vi "STORE_OUTPUT.vi"(9 "CURRENT_YEAR_DATA":string, 10 "ECODE 2":string, 11 "connection reference":T1) -> ()   [LabVIEW 2015]
uses:
  Controls/ITEM_CODE_CLUSTER.ctl
  <vilib>/addons/database/Connection.llb/Conn ObjectReference.ctl
  <vilib>/Utility/miscctls.llb/LVRowAndColumnUnsignedTypeDef.ctl
  Controls/STORE_OUTPUT_NO_CLUSTER.ctl
  Controls/ITEM_INFORMATION_CLUSTER.ctl
  Controls/Print_Data.ctl
  <vilib>/addons/database/Connection.llb/Conn Execute.vi
  <vilib>/addons/database/Recordset.llb/Rec Destroy - Connection.vi
  <vilib>/addons/database/_DB Variant To Data/Database Variant To Data.xnode
  <vilib>/addons/database/NI_Database_API.lvlib
  <vilib>/addons/database/Connection.llb/DB Tools Open Connec (String).vi
panel:
  in  "BALANCE_PRINT":bool
  in  "Print Button":bool
  out "FIFO_ARRAY":T2[](array[typedef])
  out "Location":string
  out "Lot Maker":string
  out "Maker Code":string
  out "Invoice Date":timestamp format="%<%d/%m/%Y>T"
  out "Invoice No.":string
  in  "Excle Path":path
  in  "BUTTON_EXIT":bool
  in  "BUTTON_INPUT":bool
  out "Unit 2":string
  in  "Quantity (F2)":dbl
  out "Item Code":string
  out "FIFO":string
  in  "QR Code (F3)":string
  out "Maker":string
  out "Part Name":string
  out "Product":string
  out "ECODE":string
  in  "Output Date":timestamp format="%<%d/%m/%Y>T"
  out "Output No.":string
  out "Table":string[][](table)
  # "OUTPUT MATERIAL"
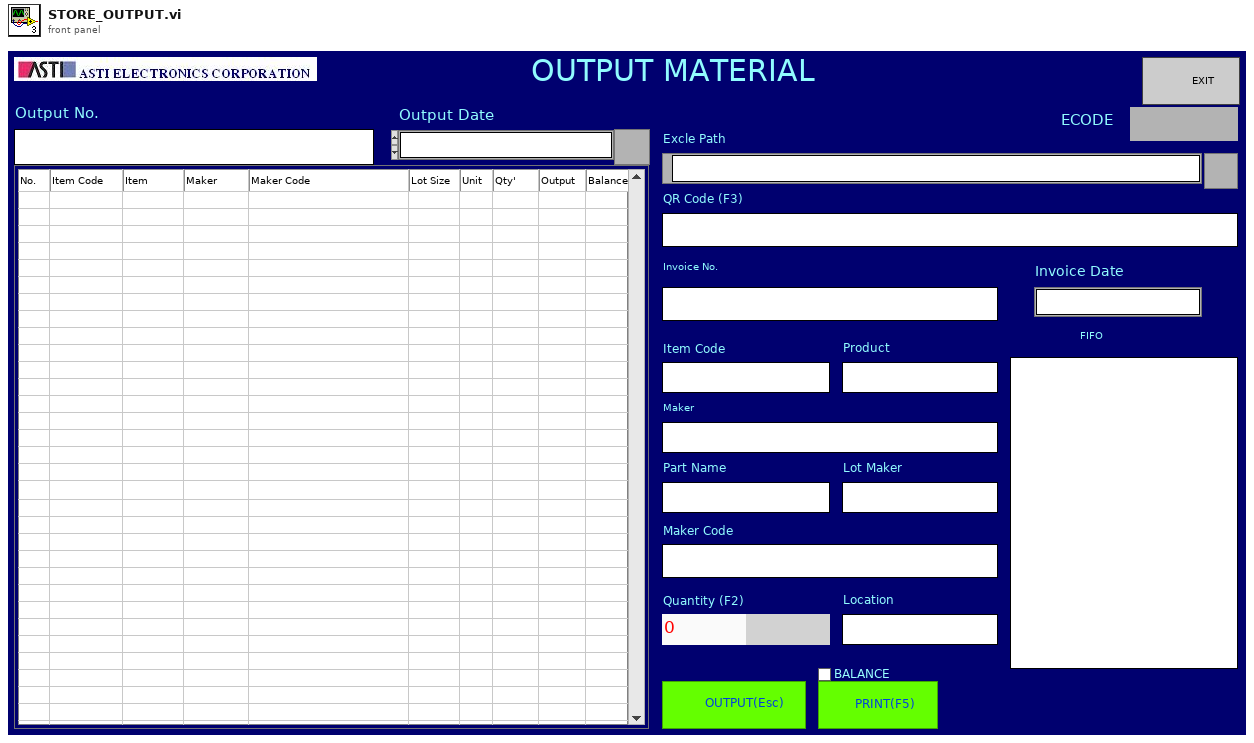
[diagram p1: front panel]
types:
  T1 = typedef "NI_Database_API.lvlib/Conn ObjectReference.ctl" = refnum<k1>
  T2 = typedef "ITEM_CODE_CLUSTER.ctl" = cluster{"ITEM_CODE":string, "INVOICE_NO":string, "INVOICE_DATE":timestamp, "LOT_MAKER":string, "QUANTITY":dbl, "INVOICE_ECODE":string, "INPUT_NO":string, "INPUT_DATE":timestamp, "INPUT_ECODE":string, "LINEBACK_NO":string, "LINEBACK_DATE":timestamp, "LINEBACK_ECODE":string, "OUTPUT_NO":string, "OUTPUT_DATE":timestamp, "OUTPUT_ECODE":string, "DESTINATION":string}
  T3 = typedef "LVRowAndColumnUnsignedTypeDef.ctl" = cluster{"Row":u32, "Column":u32}
  T4 = typedef "STORE_OUTPUT_NO_CLUSTER.ctl" = cluster{"NO":dbl, "ITEM_CODE":string, "ITEM":string, "MAKER":string, "MAKER_CODE":string, "LOT_SIZE":dbl, "UNIT":string, "QUANTITY":dbl, "INPUT":dbl, "BALANCE":dbl, "DESTINATION":string, "OUTPUT_NO":string}
  T5 = cluster{"start (-1, -1)":cluster{"row":i32, "column":i32}, "end (-1, -1)":cluster{"row":i32, "column":i32}}
  T6 = cluster{"OUTPUT_NO":string, "OUTPUT_DATE":timestamp, "ECODE":string}
  T7 = typedef "ITEM_INFORMATION_CLUSTER.ctl" = cluster{"PRODUCT":string, "ITEM_CODE":string, "PART_NAME":string, "MAKER":string, "PART_NO":string, "LOT_SIZE":dbl, "UNIT":string, "LENGTH-OFFSET":string, "BARCODE":string, "PROCESS":string, "INVENTORY_LOCAL":string, "TARE":dbl, "SAMPLE":dbl}
  T8 = typedef "Print_Data.ctl" = cluster{"QR_code Text":string, "Lot Maker":string, "Item Code (F3)":string, "date/time string":string, "Invoice No.":string, "Maker":string, "Part No.(F2) ":string, "Location":string, "Product":string, "Qty":string, "ECODE":string}
  T9 = typedef "NI_Database_API.lvlib/Rec ObjectReference.ctl" = refnum<k1>
  T10 = cluster{"Output No.":string, "seconds since 1Jan1904":timestamp, "ECODE":string, "DESTINATION":string}
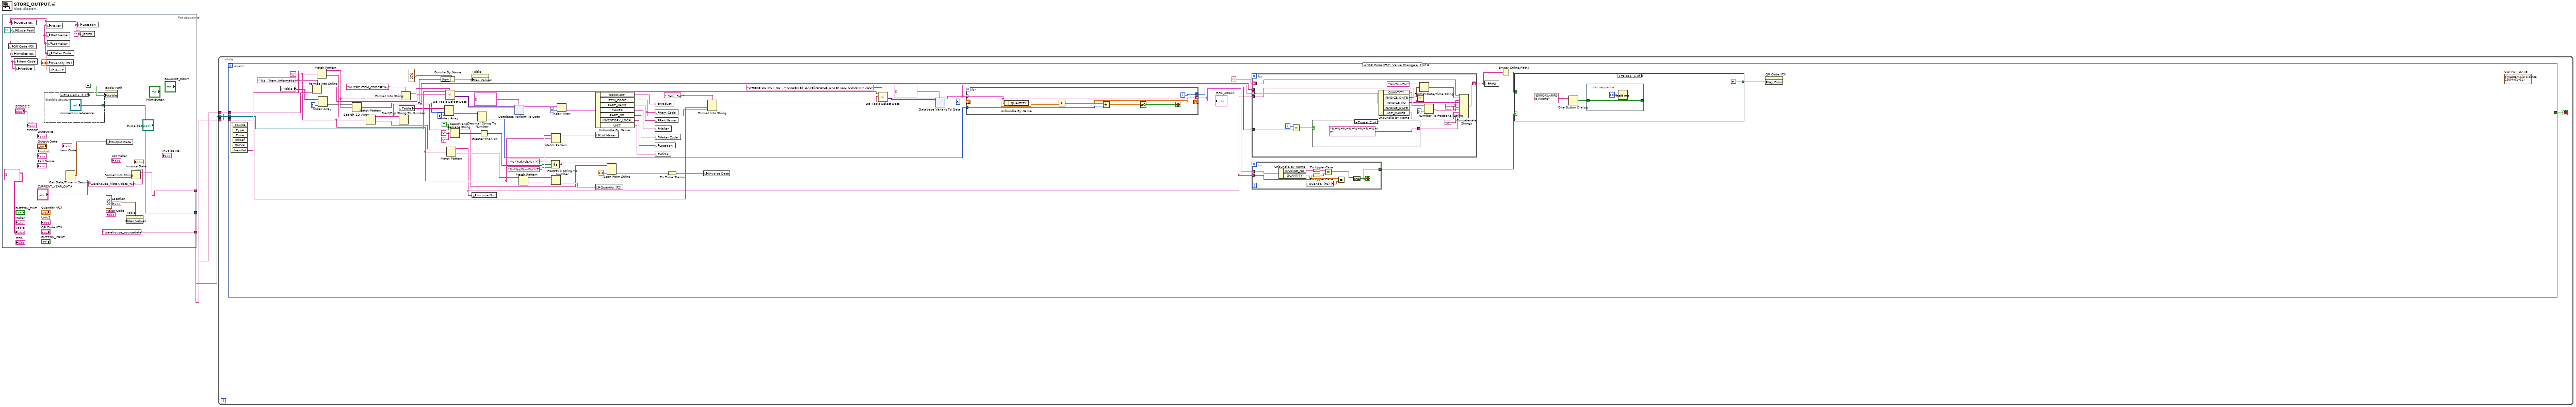
[diagram p0: block diagram]
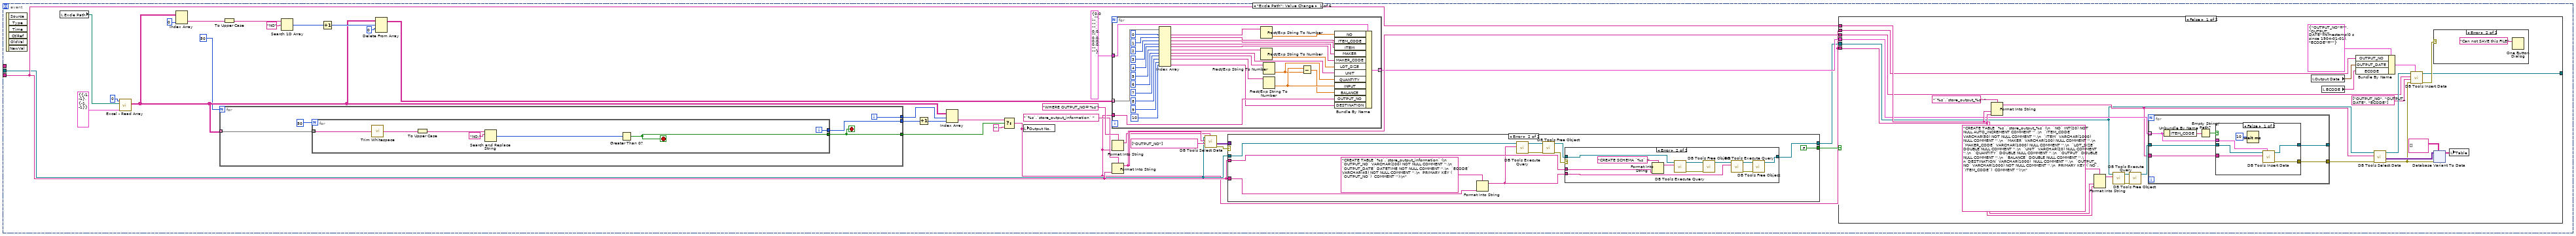
[diagram p2: hidden frame]
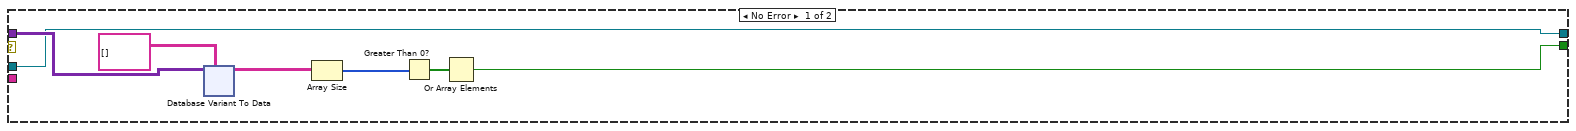
[diagram p3: hidden frame]
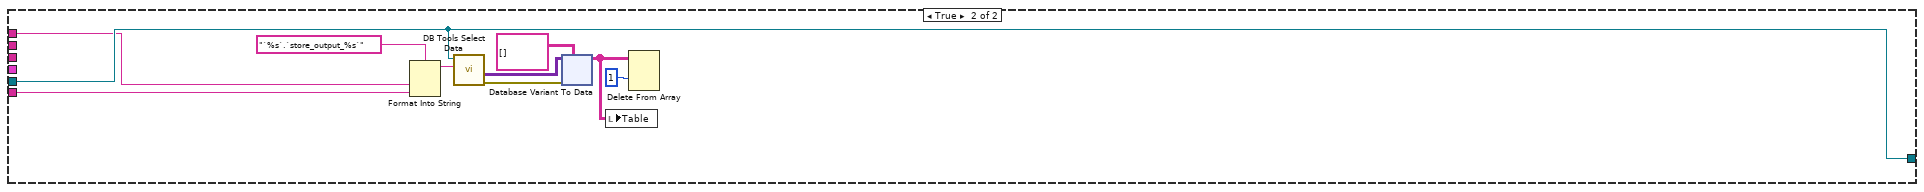
[diagram p7: hidden frame]
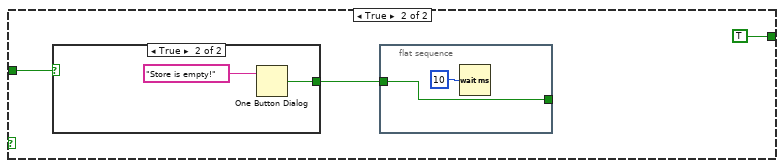
[diagram p8: hidden frame]
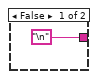
[diagram p10: hidden frame]
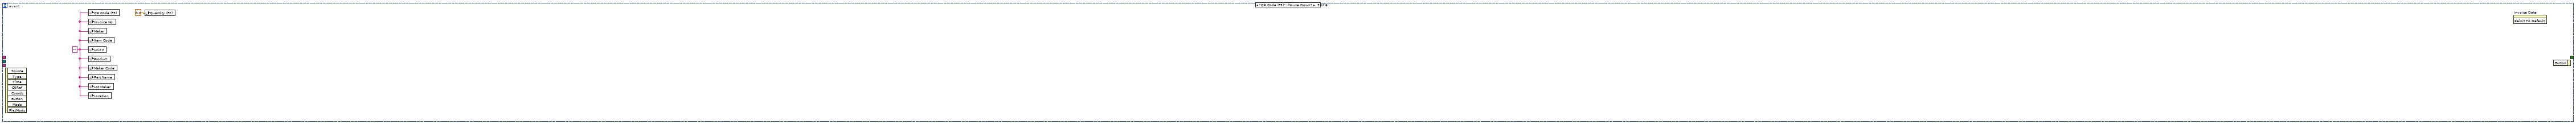
[diagram p11: hidden frame]
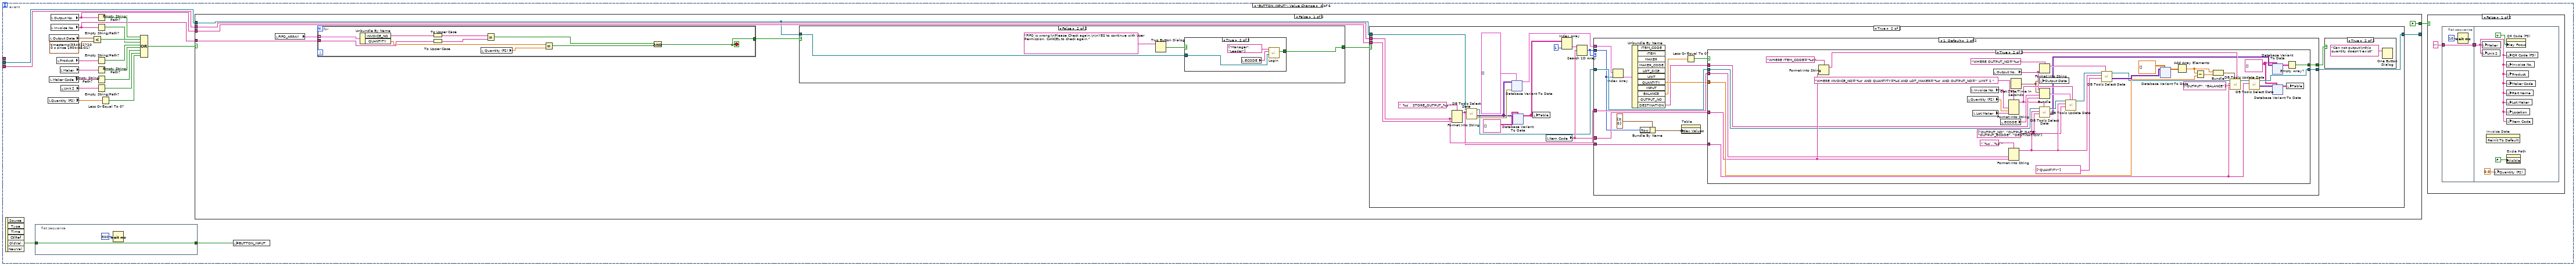
[diagram p12: hidden frame]
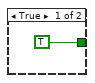
[diagram p14: hidden frame]
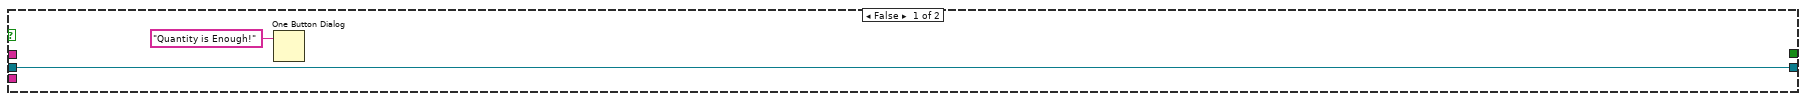
[diagram p18: hidden frame]
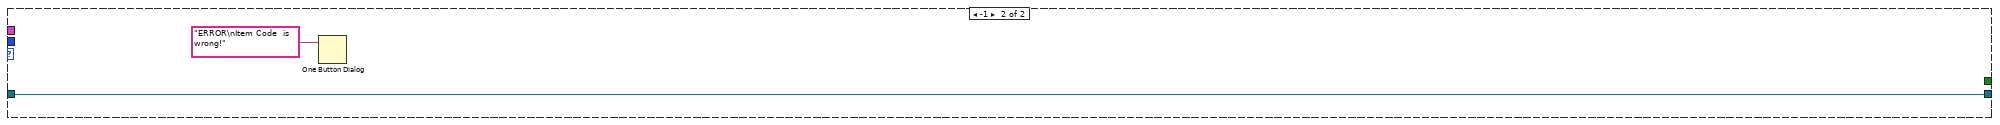
[diagram p19: hidden frame]
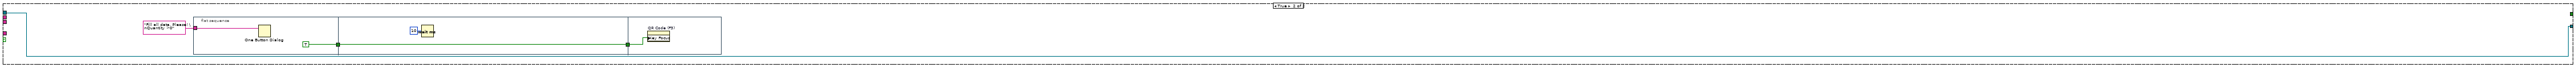
[diagram p20: hidden frame]
diagram:
  n1 = flat-sequence {
    tunnel: [w16] -> w3
    tunnel: [w14] -> w2
    tunnel: ["warehouse_sourcedata" ("table")] -> w1
    frame #0 {
      w12 = "" ("FIFO")
      n2 = local write "QR Code (F3)"(w12) -> ()
      n3 = local write "Invoice No."(w12) -> ()
      n4 = local write "Output No."(w12) -> ()
      n5 = local write "Excle Path"(path "" ("Excle Path")) -> ()
      n6 = local write "Item Code"(w12) -> ()
      n7 = local write "Product"(w12) -> ()
      n8 = disable-structure shown="Enabled" {
        disable-tunnel: [w17 "connection reference"] -> w16
        frame Disabled {
          n9 = call-poly <vilib>:"DB Tools Open Connection.vi"("password"="871994" ("userID"), "userID"="hoangbao2106", "connection information"="Database" ("userID")) -> ("connection reference"=w17:T1)  [unwired: 5 in, 1 out]
        }
        frame Enabled {
        }
      }
      n10 = local write "Maker"(w12) -> ()
      n11 = local write "Part Name"(w12) -> ()
      n12 = local write "Quantity (F2)"(0.0 ("Quantity")) -> ()
      n13 = local write "Lot Maker"(w12) -> ()
      n14 = local write "Maker Code"(w12) -> ()
      n15 = local write "Unit 2"(w12) -> ()
      n16 = Get Date/Time In Seconds() -> (seconds since 1Jan1904=w9:timestamp)
      n17 = local write "Location"(w12) -> ()
      n18 = local write "FIFO"(w12) -> ()
      n19 = property on="Excle Path" class="Path"("Visible"=TRUE) -> ()  [unwired: 2 in, 2 out]
      n20 = local write "Output Date"(w9) -> ()
      n21 = property on="Table" class="Tbl (strict)"("Index Values"=T3 {"Row"=0, "Column"=0}) -> ()  [unwired: 2 in, 2 out]
      n22 = Format Into String(format string="warehouse_historydata_%s" ("table"), "CURRENT_YEAR_DATA") -> (resulting string=w14:string)  [unwired: 2 in, 1 out]
      "Table" <- string[][] []
      "ECODE" <- "ECODE 2"
    }
  }
  n23 = while {
    tunnel: w3 -> [w24]
    tunnel: w2 -> [w23]
    tunnel: w1 -> [w22]
    stop <- w25 stop-if-true
    n24 = event shown="[1] \"QR Code (F3)\": Value Change" {
      selector: _ -> [_ _ _ _ _ _]
      dyn-events: _ -> [_ _ _ _ _ _]
      timeout: _ -> [_ _ _ _ _ _]
      tunnel: [_ _ _ _ _ TRUE] -> w25
      tunnel: w24 -> [w28 w377 _ w1411 _ _]
      tunnel: w23 -> [w29 w360 _ w1410 _ _]
      tunnel: w22 -> [_ w375 _ _ _ _]
      event "Excle Path": Value Change {
        n25 = event-data() -> ()  [unwired: 1 in, 6 out]
        n26 = local read "Excle Path"() -> (w30:path)
        n27 = call "Excel - Read Array.vi"("Cluster"=T5 {"start (-1, -1)"={"row"=-1, "column"=-1}, "end (-1, -1)"={"row"=-1, "column"=-1}}, "Path"=w30, "worksheet index (0)"=0) -> ("Element 1"=w43:string[][])  [unwired: 5 in, 1 out]
        n28 = Index Array(array=w43, index (col)=0 ("disabled index (col)")) -> (element=w41:string[])  [unwired: 1 in]
        n29 = for {
          N: 50 -> [_]
          tunnel: w43 -> [w306] mode=indexing
          tunnel: [w305] -> w36
          tunnel: [w303] -> w34
          tunnel: [w302] -> w33
          i -> [w305]
          stop <- w302 stop-if-true
          n30 = for {
            N: 50 -> [_]
            tunnel: w306 -> [w312] mode=indexing
            tunnel: [w307] -> w302
            tunnel: [w313] -> w303
            i -> [w313]
            stop <- w307 stop-if-true
            n31 = call <vilib>:"Trim Whitespace.vi"("string"=w312) -> ("trimmed string"=w311:string)  [unwired: 1 in]
            n32 = To Upper Case(1:w311) -> (0:w310:string)
            n33 = Search and Replace String(input string=w310, search string="NO:" ("y")) -> (number of replacements=w308:i32)  [unwired: 6 in, 3 out]
            n34 = Greater Than 0?(x=w308) -> (x > 0?=w307:bool)
          }
        }
        n35 = To Upper Case(1:w41) -> (0:w42:string[])
        n36 = Search 1D Array(1D array=w42, element="NO") -> (index of element=w44:i32)  [unwired: 1 in]
        n37 = Increment(x=w44) -> (x+1=w45:i32)
        n38 = Delete From Array(array=w43, length=w45, index (row)=0) -> (array with subset deleted=w55:string[][])  [unwired: 1 in, 1 out]
        n39 = Increment(x=w34) -> (x+1=w35:i32)
        n40 = Index Array(array=w43, index (row)=w36, index (col)=w35) -> (element=w37:string)
        n41 = Select(t=w37, s=w33, f="") -> (s? t:f=w27:string)
        n42 = local write "Output No."(w27) -> ()
        n43 = for {
          tunnel: w55 -> [w87] mode=indexing
          tunnel: T4 {"NO"=0.0, "ITEM_CODE"="", "ITEM"="", "MAKER"="", "MAKER_CODE"="", "LOT_SIZE"=0.0, "UNIT"="", "QUANTITY"=0.0, "INPUT"=0.0, "BALANCE"=0.0, "DESTINATION"="", "OUTPUT_NO"=""} -> [w88]
          tunnel: [w65] -> w57 mode=indexing
          tunnel: w27 -> [w64]
          n44 = Index Array(array=w87, index #1=0 ("index"), index #2=1 ("index"), index #3=2 ("index"), index #4=3 ("index"), index #5=4 ("index"), index #6=5 ("index"), index #7=6 ("index"), index #8=7 ("index"), index #9=8 ("index"), index #10=9 ("index"), index #11=10 ("index")) -> (element #1=w76:string, element #2=w74:string, element #3=w73:string, element #4=w72:string, element #5=w71:string, element #6=w70:string, element #7=w68:string, element #8=w67:string, element #9=w66:string, element #11=w59:string)  [unwired: 1 out]
          n45 = Fract/Exp String To Number(string=w76) -> (number=w75:dbl)  [unwired: 3 in, 1 out]
          n46 = Fract/Exp String To Number(string=w70) -> (number=w69:dbl)  [unwired: 3 in, 1 out]
          n47 = Fract/Exp String To Number(string=w67) -> (number=w62:dbl)  [unwired: 3 in, 1 out]
          n48 = Fract/Exp String To Number(string=w66) -> (number=w63:dbl)  [unwired: 3 in, 1 out]
          n49 = Subtract(x=w63, y=w62) -> (x-y=w61:dbl)
          n50 = Bundle By Name(cluster=w88, "NO"=w75, "ITEM_CODE"=w74, "ITEM"=w73, "MAKER"=w72, "MAKER_CODE"=w71, "LOT_SIZE"=w69, "UNIT"=w68, "QUANTITY"=w62, "INPUT"=w63, "BALANCE"=w61, "OUTPUT_NO"=w64, "DESTINATION"=w59) -> (w65:T4)
        }
        n51 = Format Into String(format string="WHERE OUTPUT_NO='%s'", w27) -> (resulting string=w49:string)  [unwired: 2 in, 1 out]
        n52 = Format Into String(format string="`%s`.`store_output_information` ", w29) -> (resulting string=w58:string)  [unwired: 2 in, 1 out]
        n53 = call <vilib>:"DB Tools Select Data.vi"("condition"=w49, "columns"=string[] ["OUTPUT_NO"], "table"=w58, "connection reference"=w28) -> ("error out"=w53:errorcluster, "data"=w50:variant[][])  [unwired: 2 in, 1 out]
        n54 = case shown="Error" w53 {
          tunnel: w50 -> [w95 _]
          tunnel: [w90 FALSE] -> w52
          tunnel: w28 -> [w89 w147]
          tunnel: [w89 w143] -> w54
          tunnel: w29 -> [_ w145]
          tunnel: w29 -> [_ w141]
          frame No Error {
            n55 = xnode "Database Variant To Data"("database variant"=w95, "type"=string[][] []) -> ("data"=w93:string[][])  [unwired: 1 in, 1 out]
            n56 = Array Size(array=w93) -> (size(s)=w92:i32[])
            n57 = Greater Than 0?(x=w92) -> (x > 0?=w91:bool[])
            n58 = Or Array Elements(Boolean array=w91) -> (logical OR=w90:bool)
          }
          frame Error {
            n59 = Format Into String(format string="CREATE TABLE `%s`.`store_output_information` (\n  `OUTPUT_NO` VARCHAR(200) NOT NULL COMMENT '',\n  `OUTPUT_DATE` DATETIME NOT NULL COMMENT '',\n  `ECODE` VARCHAR(45) NOT NULL COMMENT '',\n  PRIMARY KEY (  `OUTPUT_NO`)  COMMENT '');\n", w141) -> (resulting string=w140:string)  [unwired: 2 in, 1 out]
            n60 = call-poly <vilib>:"DB Tools Execute Query.vi"("SQL query"=w140, "connection reference"=w147) -> ("error out"=w149:errorcluster, "recordset reference"=w150:T9)  [unwired: 6 in]
            n61 = call-poly <vilib>:"DB Tools Free Object.vi"("error in (no error)"=w149, "recordset reference"=w150) -> ("error out"=w146:errorcluster, "connection reference"=w144:T1)  [unwired: 8 in]
            n62 = case shown="Error" w146 {
              tunnel: w144 -> [w151 w162]
              tunnel: w145 -> [_ w160]
              tunnel: w140 -> [_ w154]
              tunnel: [w151 w153] -> w143
              frame No Error {
              }
              frame Error {
                n63 = Format Into String(format string="CREATE SCHEMA `%s` ;" ("SQL query"), w160) -> (resulting string=w152:string)  [unwired: 2 in, 1 out]
                n64 = call-poly <vilib>:"DB Tools Execute Query.vi"("SQL query"=w152, "connection reference"=w162) -> ("error out"=w158:errorcluster, "recordset reference"=w159:T9)  [unwired: 6 in]
                n65 = call-poly <vilib>:"DB Tools Free Object.vi"("error in (no error)"=w158, "recordset reference"=w159) -> ("connection reference"=w155:T1)  [unwired: 8 in, 1 out]
                n66 = call-poly <vilib>:"DB Tools Execute Query.vi"("SQL query"=w154, "connection reference"=w155) -> ("error out"=w157:errorcluster, "recordset reference"=w156:T9)  [unwired: 6 in]
                n67 = call-poly <vilib>:"DB Tools Free Object.vi"("error in (no error)"=w157, "recordset reference"=w156) -> ("connection reference"=w153:T1)  [unwired: 8 in, 1 out]
              }
            }
          }
        }
        n68 = case shown="False" w52 {
          tunnel: w54 -> [w163 w257]
          tunnel: w29 -> [w184 w251]
          tunnel: w27 -> [w183 w252]
          tunnel: [w170 w257] -> _
          tunnel: w57 -> [w182 _]
          tunnel: w58 -> [w173 _]
          tunnel: w27 -> [w168 _]
          frame False {
            n69 = Format Into String(format string="`%s`.`store_output_%s` " ("SQL query"), w184, w183) -> (resulting string=w177:string)  [unwired: 2 in, 1 out]
            n70 = Format Into String(format string="CREATE TABLE `%s`.`store_output_%s` (\n  `NO` INT(20) NOT NULL AUTO_INCREMENT COMMENT '' ,\n  `ITEM_CODE` VARCHAR(50) NOT NULL COMMENT '',\n  `ITEM` VARCHAR(1000) NULL COMMENT '',\n  `MAKER` VARCHAR(100) NULL COMMENT '',\n  `MAKER_CODE` VARCHAR(1000) NULL COMMENT '',\n  `LOT_SIZE` DOUBLE NULL COMMENT '',\n  `UNIT` VARCHAR(20) NULL COMMENT '',\n  `QUANTITY` DOUBLE NULL COMMENT '',\n  `OUTPUT` DOUBLE NULL COMMENT '',\n  `BALANCE` DOUBLE NULL COMMENT '',\n`DESTINATION` VARCHAR(1000)  NULL COMMENT '',\n  `OUTPUT_NO` VARCHAR(1000) NOT NULL COMMENT '',\n  PRIMARY KEY (`NO`, `ITEM_CODE`)  COMMENT '');\n" ("SQL query"), w184, w183) -> (resulting string=w176:string)  [unwired: 2 in, 1 out]
            n71 = call-poly <vilib>:"DB Tools Execute Query.vi"("SQL query"=w176, "connection reference"=w163) -> ("error out"=w186:errorcluster, "recordset reference"=w187:T9)  [unwired: 6 in]
            n72 = call-poly <vilib>:"DB Tools Free Object.vi"("error in (no error)"=w186, "recordset reference"=w187) -> ("connection reference"=w178:T1)  [unwired: 8 in, 1 out]
            n73 = for {
              tunnel: w178 -> [w240]
              tunnel: w177 -> [w239]
              tunnel: w182 -> [w236] mode=indexing
              tunnel: [w238] -> _
              tunnel: [w237] -> w175
              n74 = Unbundle By Name(w236) -> ("ITEM_CODE"=w235:string)
              n75 = Empty String/Path?(string/path=w235) -> (empty?=w234:bool)
              n76 = case shown="False" w234 {
                tunnel: w240 -> [w246 w247]
                tunnel: w239 -> [w245 _]
                tunnel: w236 -> [w244 _]
                tunnel: [w243 w247] -> w238
                tunnel: [w242 _] -> w237
                frame False {
                  n77 = Wait (ms)(milliseconds to wait=u32 10) -> ()  [unwired: 1 out]
                  n78 = call <vilib>:"DB Tools Insert Data.vi"("data"=w244, "table"=w245, "connection reference"=w246) -> ("error out"=w242:errorcluster, "connection reference out"=w243:T1)  [unwired: 7 in]
                }
                frame True {
                }
              }
            }
            n79 = local read "Output Date"() -> (w167:timestamp)
            n80 = local read "ECODE"() -> (w166:string)
            n81 = Bundle By Name(cluster=T6 {"OUTPUT_NO"="", "OUTPUT_DATE"=timestamp(0 s since 1904-01-01), "ECODE"=""}, "OUTPUT_NO"=w168, "OUTPUT_DATE"=w167, "ECODE"=w166) -> (w165:T6)
            n82 = call <vilib>:"DB Tools Select Data.vi"("error in (no error)"=w175, "table"=w177, "connection reference"=w163) -> ("error out"=w172:errorcluster, "data"=w181:variant[][], "connection reference out"=w174:T1)  [unwired: 3 in]
            n83 = call <vilib>:"DB Tools Insert Data.vi"("data"=w165, "error in (no error)"=w172, "columns"=string[] ["OUTPUT_NO", "OUTPUT_DATE", "ECODE"], "table"=w173, "connection reference"=w174) -> ("error out"=w171:errorcluster, "connection reference out"=w170:T1)  [unwired: 5 in]
            n84 = case shown="Error" w171 {
              frame No Error {
              }
              frame Error {
                n85 = One Button Dialog(message="Can not SAVE this FILE") -> ()  [unwired: 1 in, 1 out]
              }
            }
            n86 = xnode "Database Variant To Data"("database variant"=w181, "error in (no error)"=w172, "type"=string[][] []) -> ("data"=w179:string[][])  [unwired: 1 out]
            n87 = local write "Table"(w179) -> ()
          }
          frame True {
            n88 = Format Into String(format string="`%s`.`store_output_%s`", w251, w252) -> (resulting string=w250:string)  [unwired: 2 in, 1 out]
            n89 = call <vilib>:"DB Tools Select Data.vi"("table"=w250, "connection reference"=w257) -> ("error out"=w254:errorcluster, "data"=w256:variant[][])  [unwired: 4 in, 1 out]
            n90 = xnode "Database Variant To Data"("database variant"=w256, "error in (no error)"=w254, "type"=string[][] []) -> ("data"=w249:string[][])  [unwired: 1 out]
            n91 = local write "Table"(w249) -> ()
            n92 = Delete From Array(array=w249, index (row)=1) -> ()  [unwired: 2 in, 2 out]
          }
        }
      }
      event "QR Code (F3)": Value Change {
        (unwired) timestamp(0 s since 1904-01-01)  # OUTPUT_DATE
        w347 = "\\" ("regular expression")
        n93 = event-data() -> ("NewVal"=w381:string)  [unwired: 1 in, 5 out]
        n94 = local read "Table"() -> (w328:string[][])
        n95 = Format Into String(format string="`%s`.`item_information`", w375) -> (resulting string=w374:string)  [unwired: 2 in, 1 out]
        n96 = Match Pattern(string=w381, regular expression=w347) -> (before substring=w325:string, after substring=w380:string)  [unwired: 1 in, 2 out]
        n97 = Index Array(array=w328, index (col)=1 ("disabled index (col)")) -> (element=w326:string[])  [unwired: 1 in]
        n98 = Search 1D Array(1D array=w326, element=w325) -> (index of element=w321:i32)  [unwired: 1 in]
        n99 = Match Pattern(string=w380, regular expression=w347) -> (before substring=w343:string, after substring=w379:string)  [unwired: 1 in, 2 out]
        n100 = local read "Table"() -> (w322:string[][])
        n101 = Fract/Exp String To Number(string=w343) -> ()  [unwired: 3 in, 2 out]
        n102 = Format Into String(format string="WHERE ITEM_CODE='%s'", w325) -> (resulting string=w372:string)  [unwired: 2 in, 1 out]
        n103 = Bundle By Name(cluster=T3 {"Row"=0, "Column"=0} ("Index Values"), "Row"=w321) -> (w329:T3)
        n104 = Index Array(array=w322, index (row)=w321, index (col)=9 ("disabled index (col)")) -> (element=w319:string)
        n105 = call <vilib>:"DB Tools Select Data.vi"("condition"=w372, "table"=w374, "connection reference"=w377) -> ("data"=w371:variant[][], "connection reference out"=w361:T1)  [unwired: 3 in, 1 out]
        n106 = Match Pattern(string=w379, regular expression=w347) -> (before substring=w315:string, after substring=w350:string)  [unwired: 1 in, 2 out]
        n107 = Search and Replace String(replace all?=TRUE ("replace all? (F)"), input string=w343, search string="-", replace string="/" ("replace string (\"\")")) -> (result string=w332:string, number of replacements=w339:i32)  [unwired: 4 in, 2 out]
        n108 = property on="Table" class="Tbl (strict)"("Index Values"=w329) -> ()  [unwired: 2 in, 2 out]
        n109 = local write "Invoice No."(w315) -> ()
        n110 = Decimal String To Number(string=w319) -> (number=w318:i32)  [unwired: 2 in, 1 out]
        n111 = Greater Than 0?(x=w339) -> (x > 0?=w338:bool)
        n112 = xnode "Database Variant To Data"("database variant"=w371, "type"=T7[] []) -> ("data"=w369:T7[])  [unwired: 1 in, 1 out]
        n113 = Match Pattern(string=w350, regular expression=w347) -> (before substring=w349:string, after substring=w348:string)  [unwired: 1 in, 2 out]
        n114 = Select(t="%<%d/%b/%Y>T" ("format string"), s=w338, f="%<%d/%m/%Y>T" ("format string")) -> (s? t:f=w333:string)
        n115 = Match Pattern(string=w348, regular expression=w347) -> (before substring=w346:string)  [unwired: 1 in, 3 out]
        n116 = Fract/Exp String To Number(string=w349) -> (number=w378:dbl)  [unwired: 3 in, 1 out]
        n117 = Index Array(array=w369, index=0) -> (element=w367:T7)
        n118 = Unbundle By Name(w367) -> ("PRODUCT"=w366:string, "ITEM_CODE"=w358:string, "PART_NAME"=w365:string, "MAKER"=w364:string, "PART_NO"=w362:string, "INVENTORY_LOCAL"=w354:string, "UNIT"=w363:string)
        n119 = local write "Lot Maker"(w346) -> ()
        n120 = local write "Quantity (F2)"(w378) -> ()
        n121 = Scan From String(format string=w333, input string=w332, default 1=0.0) -> (output 1=w335:dbl)  [unwired: 2 in, 3 out]
        n122 = local write "Product"(w366) -> ()
        n123 = local write "Item Code"(w358) -> ()
        n124 = local write "Part Name"(w365) -> ()
        n125 = local write "Maker"(w364) -> ()
        n126 = local write "Maker Code"(w362) -> ()
        n127 = local write "Location"(w354) -> ()
        n128 = local write "Unit 2"(w363) -> ()
        n129 = To Time Stamp(1:w335) -> (0:w331:timestamp)
        n130 = local write "Invoice Date"(w331) -> ()
        n131 = Format Into String(format string="`%s`.`%s`", w360, w358) -> (resulting string=w357:string)  [unwired: 2 in, 1 out]
        n132 = call <vilib>:"DB Tools Select Data.vi"("condition"="WHERE OUTPUT_NO ='' ORDER BY DATE(INVOICE_DATE) ASC, QUANTITY ASC" ("format string"), "table"=w357, "connection reference"=w361) -> ("data"=w356:variant[][])  [unwired: 3 in, 2 out]
        n133 = xnode "Database Variant To Data"("database variant"=w356, "type"=T2[] []) -> ("data"=w324:T2[])  [unwired: 1 in, 1 out]
        n134 = for {
          tunnel: w324 -> [w392] mode=indexing
          shift-right: [w397] -> _
          shift-left: 0 -> [w398]
          tunnel: w318 -> [w396]
          tunnel: [w393] -> w317
          tunnel: [w392] -> w316 mode=indexing
          i -> [w393]
          stop <- w394 stop-if-true
          n135 = Unbundle By Name(w392) -> ("QUANTITY"=w399:dbl)
          n136 = Add(x=w399, y=w398) -> (x+y=w397:dbl)
          n137 = Add(x=w397, y=w396) -> (x+y=w395:dbl)
          n138 = Greater Or Equal To 0?(x=w395) -> (x >= 0?=w394:bool)
        }
        "FIFO_ARRAY" <- w316
        n139 = for {
          tunnel: w324 -> [w429] mode=indexing
          tunnel: w315 -> [w428]
          shift-right: [w420] -> w351
          shift-left: "" -> [w419]
          tunnel: w343 -> [_]
          tunnel: w317 -> [w416]
          i -> [w414]
          w418 = "\\" ("string")
          n140 = Equal?(x=w414, y=w416) -> (x = y?=w415:bool)
          n141 = case shown="True" w415 {
            tunnel: ["\n" "%~%~%~%~%~%~%~%~\n"] -> w412
            frame False {
            }
            frame True {
            }
          }
          n142 = Unbundle By Name(w429) -> ("QUANTITY"=w425:dbl, "INVOICE_DATE"=w427:timestamp, "INVOICE_NO"=w422:string, "LOT_MAKER"=w417:string)  [unwired: 1 out]
          n143 = Equal?(x=w428, y=w422) -> ()  [unwired: 1 out]
          n144 = Format Date/Time String(time format string (%c)="%d/%m/%Y", seconds (now)=w427) -> (date/time string=w423:string)  [unwired: 1 in]
          n145 = Number To Fractional String(number=w425, precision (6)=i16 0) -> (F-format string=w421:string)  [unwired: 2 in]
          n146 = Concatenate Strings(w419, w423, w418, w422, w418, w421, w418, w417, "\n", w412) -> (w420:string)
        }
        n147 = for {
          tunnel: w316 -> [w391] mode=indexing
          tunnel: w315 -> [w388]
          tunnel: [w383] -> w314
          stop <- w383 stop-if-true
          n148 = Unbundle By Name(w391) -> ("INVOICE_NO"=w387:string, "QUANTITY"=w385:dbl)
          n149 = local read "Quantity (F2)"() -> (w386:dbl)
          n150 = To Upper Case(1:w387) -> (0:w389:string)
          n151 = To Upper Case(1:w388) -> (0:w390:string)
          n152 = Equal?(x=w389, y=w390) -> (x = y?=w382:bool)
          n153 = Equal?(x=w385, y=w386) -> (x = y?=w384:bool)
          n154 = And(x=w382, y=w384) -> (x .and. y?=w383:bool)
        }
        n155 = local write "FIFO"(w351) -> ()
        n156 = Empty String/Path?(string/path=w351) -> (empty?=w345:bool)
        n157 = case shown="False" w314 {
          tunnel: w345 -> [_ w407]
          tunnel: [TRUE ("Key Focus") TRUE ("Key Focus")] -> w344
          frame False {
            n158 = One Button Dialog(message="ERROR!\nFIFO is Wrong") -> (true=w401:bool)  [unwired: 1 in]
            n159 = flat-sequence {
              tunnel: w401 -> [w403]
              tunnel: [w403] -> _
              frame #0 {
                n160 = Wait (ms)(milliseconds to wait=u32 10) -> ()  [unwired: 1 out]
              }
            }
          }
          frame True {
            n161 = case shown="True" w407 {
              tunnel: [_ w410] -> w405
              frame False {
              }
              frame True {
                n162 = One Button Dialog(message="Store is empty!") -> (true=w410:bool)  [unwired: 1 in]
              }
            }
            n163 = flat-sequence {
              tunnel: [w409] -> _
              tunnel: w405 -> [w409]
              frame #0 {
                n164 = Wait (ms)(milliseconds to wait=u32 10) -> ()  [unwired: 1 out]
              }
            }
          }
        }
        n165 = property on="QR Code (F3)" class="Str"("Key Focus"=w344) -> ()  [unwired: 2 in, 2 out]
      }
      event "QR Code (F3)": Mouse Down? {
        w1404 = ""
        n166 = event-data() -> ()  [unwired: 1 in, 8 out]
        n167 = local write "QR Code (F3)"(w1404) -> ()
        n168 = local write "Invoice No."(w1404) -> ()
        n169 = local write "Maker"(w1404) -> ()
        n170 = local write "Item Code"(w1404) -> ()
        n171 = local write "Unit 2"(w1404) -> ()
        n172 = local write "Product"(w1404) -> ()
        n173 = local write "Maker Code"(w1404) -> ()
        n174 = local write "Part Name"(w1404) -> ()
        n175 = local write "Lot Maker"(w1404) -> ()
        n176 = local write "Location"(w1404) -> ()
        n177 = local write "Quantity (F2)"(0.0 ("Quantity")) -> ()
        n178 = invoke on="Invoice Date" class="AbsTime (strict)" method="Reinit To Default"() -> ()  [unwired: 3 in, 3 out]
        n179 = event-data() -> ()  [unwired: 2 in, 1 out]
      }
      event "BUTTON_INPUT": Value Change {
        n180 = event-data() -> ("OldVal"=w1405:bool)  [unwired: 1 in, 5 out]
        n181 = flat-sequence {
          tunnel: [w1429] -> w1406
          tunnel: w1405 -> [w1429]
          frame #0 {
            n182 = Wait (ms)(milliseconds to wait=u32 500) -> ()  [unwired: 1 out]
          }
        }
        n183 = local read "Quantity (F2)"() -> (w1419:dbl)
        n184 = local read "Output Date"() -> (w1427:timestamp)
        n185 = local read "Maker Code"() -> (w1421:string)
        n186 = local read "Output No."() -> (w1409:string)
        n187 = local read "Invoice No."() -> (w1407:string)
        n188 = local read "Product"() -> (w1423:string)
        n189 = local read "Maker"() -> (w1422:string)
        n190 = local read "Unit 2"() -> (w1420:string)
        n191 = Less?(x=w1427, y=timestamp(3345127200 s since 1904-01-01)) -> (x < y?=w1424:bool)
        n192 = Empty String/Path?(string/path=w1409) -> (empty?=w1425:bool)
        n193 = Empty String/Path?(string/path=w1407) -> (empty?=w1418:bool)
        n194 = Empty String/Path?(string/path=w1423) -> (empty?=w1417:bool)
        n195 = Empty String/Path?(string/path=w1422) -> (empty?=w1416:bool)
        n196 = Empty String/Path?(string/path=w1421) -> (empty?=w1415:bool)
        n197 = Empty String/Path?(string/path=w1420) -> (empty?=w1414:bool)
        n198 = Less Or Equal To 0?(x=w1419) -> (x <= 0?=w1413:bool)
        n199 = Compound Arithmetic op=OR(w1425, w1424, w1418, w1417, w1416, w1415, w1414, w1413) -> (w1412:bool)
        n200 = case shown="False" w1412 {
          tunnel: w1411 -> [w1439 w2106]
          tunnel: w1410 -> [w1445 _]
          tunnel: w1409 -> [w1446 _]
          tunnel: [w1444 w2106] -> _
          tunnel: [FALSE _] -> w1408
          tunnel: w1407 -> [w1442 _]
          frame False {
            n201 = local read "FIFO_ARRAY"() -> (w1438:T2[])
            n202 = for {
              tunnel: w1442 -> [w1456]
              tunnel: [w1447] -> w1440
              tunnel: w1438 -> [w1452] mode=indexing
              stop <- w1447 stop-if-true
              n203 = Unbundle By Name(w1452) -> ("INVOICE_NO"=w1455:string, "QUANTITY"=w1450:dbl)
              n204 = To Upper Case(1:w1455) -> (0:w1454:string)
              n205 = To Upper Case(1:w1456) -> (0:w1453:string)
              n206 = local read "Quantity (F2)"() -> (w1451:dbl)
              n207 = Equal?(x=w1454, y=w1453) -> (x = y?=w1449:bool)
              n208 = Equal?(x=w1450, y=w1451) -> (x = y?=w1448:bool)
              n209 = And(x=w1449, y=w1448) -> (x .and. y?=w1447:bool)
            }
            n210 = case shown="False" w1440 {
              tunnel: [TRUE w1458] -> w1441
              tunnel: w1439 -> [_ w1459]
              frame True {
              }
              frame False {
                n211 = Two Button Dialog(message="FIFO is wrong!\nPlease Check again.\n\nYES to continue with User Permission, CANCEL to check again.") -> (T button?=w1460:bool)  [unwired: 2 in]
                n212 = case shown="True" w1460 {
                  tunnel: w1459 -> [_ w1465]
                  tunnel: [_ w1462] -> w1458
                  frame False {
                  }
                  frame True {
                    n213 = local read "ECODE"() -> (w1464:string)
                    n214 = call "Login.vi"("connection reference"=w1465, "ACCOUNT:"=w1464, "Permission"=string[] ["Manager", "Leader"]) -> ("OK"=w1462:bool)  [unwired: 7 in, 1 out]
                  }
                }
              }
            }
            n215 = case shown="True" w1441 {
              tunnel: w1439 -> [w1466 w1479]
              tunnel: w1446 -> [_ w1478]
              tunnel: w1445 -> [_ w1473]
              tunnel: [w1466 w1470] -> w1444
              frame False {
              }
              frame True {
                n216 = Format Into String(format string="`%s`.`STORE_OUTPUT_%s`", w1473, w1478) -> (resulting string=w1471:string)  [unwired: 2 in, 1 out]
                n217 = call <vilib>:"DB Tools Select Data.vi"("table"=w1471, "connection reference"=w1479) -> ("error out"=w1484:errorcluster, "data"=w1482:variant[][], "connection reference out"=w1468:T1)  [unwired: 4 in]
                n218 = xnode "Database Variant To Data"("database variant"=w1482, "error in (no error)"=w1484, "type"=T4[] []) -> ("data"=w1474:T4[])  [unwired: 1 out]
                n219 = xnode "Database Variant To Data"("database variant"=w1482, "type"=string[][] []) -> ("data"=w1475:string[][])  [unwired: 1 in, 1 out]
                n220 = local write "Table"(w1475) -> ()
                n221 = local read "Item Code"() -> (w1472:string)
                n222 = Index Array(array=w1475, index (col)=1 ("disabled index (col)")) -> (element=w1477:string[])  [unwired: 1 in]
                n223 = Search 1D Array(1D array=w1477, element=w1472) -> (index of element=w1467:i32)  [unwired: 1 in]
                n224 = case shown="1, Default" w1467 {
                  tunnel: w1474 -> [w1500 _]
                  tunnel: w1468 -> [w1494 w1677]
                  tunnel: w1473 -> [w1493 _]
                  tunnel: w1472 -> [w1492 _]
                  tunnel: w1471 -> [w1490 _]
                  tunnel: [w1489 w1677] -> w1470
                  tunnel: [w1488 _] -> w1469
                  tunnel: w1467 -> [w1486 _]
                  frame 1, Default {
                    n225 = Index Array(array=w1500, index=w1486) -> (element=w1497:T4)
                    n226 = Unbundle By Name(w1497) -> ("QUANTITY"=w1491:dbl, "BALANCE"=w1496:dbl, "DESTINATION"=w1487:string)  [unwired: 8 out]
                    n227 = Bundle By Name(cluster=T3 {"Row"=0, "Column"=0} ("Index Values"), "Row"=w1486) -> (w1498:T3)
                    n228 = property on="Table" class="Tbl (strict)"("Index Values"=w1498) -> ()  [unwired: 2 in, 2 out]
                    n229 = Less Or Equal To 0?(x=w1496) -> (x <= 0?=w1495:bool)
                    n230 = case shown="True" w1495 {
                      tunnel: w1494 -> [w1502 w1514]
                      tunnel: w1493 -> [_ w1542]
                      tunnel: w1492 -> [_ w1522]
                      tunnel: w1491 -> [_ w1529]
                      tunnel: w1490 -> [_ w1519]
                      tunnel: [w1502 w1516] -> w1489
                      tunnel: [_ w1506] -> w1488
                      tunnel: w1487 -> [_ w1504]
                      frame False {
                        n231 = One Button Dialog(message="Quantity is Enough!") -> ()  [unwired: 1 in, 1 out]
                      }
                      frame True {
                        w1508 = string[][] []
                        w1510 = string[] ["OUTPUT_NO", "OUTPUT_DATE", "OUTPUT_ECODE", "DESTINATION"] ("columns")
                        n232 = Format Into String(format string="WHERE ITEM_CODE='%s'" ("condition"), w1522) -> (resulting string=w1515:string)  [unwired: 2 in, 1 out]
                        n233 = local read "Quantity (F2)"() -> (w1537:dbl)
                        n234 = local read "Invoice No."() -> (w1538:string)
                        n235 = local read "Lot Maker"() -> (w1503:string)
                        n236 = local read "Output No."() -> (w1534:string)
                        n237 = local read "ECODE"() -> (w1539:string)
                        n238 = Format Into String(format string="WHERE INVOICE_NO='%s' AND QUANTITY=%d AND LOT_MAKER='%s' AND OUTPUT_NO='' LIMIT 1 ", w1538, w1537, w1503) -> (resulting string=w1511:string)  [unwired: 2 in, 1 out]
                        n239 = Format Into String(format string="`%s`.`%s`", w1542, w1522) -> (resulting string=w1513:string)  [unwired: 2 in, 1 out]
                        n240 = Get Date/Time In Seconds() -> (seconds since 1Jan1904=w1505:timestamp)
                        n241 = Format Into String(format string="WHERE OUTPUT_NO='%s'" ("condition"), w1534) -> (resulting string=w1533:string)  [unwired: 2 in, 1 out]
                        n242 = local write "Output Date"(w1505) -> ()
                        n243 = Bundle("Output No."=w1534, "seconds since 1Jan1904"=w1505, "ECODE"=w1539, "DESTINATION"=w1504) -> (w1541:T10)  [unwired: 1 in]
                        n244 = call <vilib>:"DB Tools Select Data.vi"("condition"=w1511, "columns"=w1510, "table"=w1513, "connection reference"=w1514) -> ("data"=w1509:variant[][], "connection reference out"=w1512:T1)  [unwired: 2 in, 1 out]
                        n245 = call <vilib>:"DB Tools Update Data.vi"("condition"=w1511, "data"=w1541, "columns"=w1510, "table"=w1513, "connection reference"=w1512) -> ("connection reference out"=w1525:T1)  [unwired: 5 in, 1 out]
                        n246 = call <vilib>:"DB Tools Select Data.vi"("condition"=w1533, "columns"=string[] ["QUANTITY"], "table"=w1513, "connection reference"=w1525) -> ("data"=w1531:variant[][], "connection reference out"=w1526:T1)  [unwired: 2 in, 1 out]
                        n247 = xnode "Database Variant To Data"("database variant"=w1531, "type"=dbl[][] []) -> ("data"=w1530:dbl[][])  [unwired: 1 in, 1 out]
                        n248 = Add Array Elements(numeric array=w1530) -> (sum=w1528:dbl)
                        n249 = Subtract(x=w1528, y=w1529) -> (x-y=w1527:dbl)
                        n250 = Bundle(w1528, w1527) -> (w1524:cluster{dbl, dbl})  [unwired: 1 in]
                        n251 = call <vilib>:"DB Tools Update Data.vi"("condition"=w1515, "data"=w1524, "columns"=string[] ["OUTPUT", "BALANCE"], "table"=w1519, "connection reference"=w1526) -> ("connection reference out"=w1520:T1)  [unwired: 5 in, 1 out]
                        n252 = call <vilib>:"DB Tools Select Data.vi"("table"=w1519, "connection reference"=w1520) -> ("data"=w1517:variant[][], "connection reference out"=w1516:T1)  [unwired: 4 in, 1 out]
                        n253 = xnode "Database Variant To Data"("database variant"=w1509, "type"=w1508) -> ("data"=w1507:string[][])  [unwired: 1 in, 1 out]
                        n254 = xnode "Database Variant To Data"("database variant"=w1517, "type"=w1508) -> ("data"=w1518:string[][])  [unwired: 1 in, 1 out]
                        n255 = local write "Table"(w1518) -> ()
                        n256 = Empty Array?(array=w1507) -> (empty?=w1506:bool)
                      }
                    }
                  }
                  frame -1 {
                    n257 = One Button Dialog(message="ERROR\nItem Code  is wrong!") -> ()  [unwired: 1 in, 1 out]
                  }
                }
                n258 = case shown="True" w1469 {
                  frame False {
                  }
                  frame True {
                    n259 = One Button Dialog(message="Can not output!\nthis quantity doesn't exist") -> ()  [unwired: 1 in, 1 out]
                  }
                }
              }
            }
          }
          frame True {
            n260 = flat-sequence {
              tunnel: "Fill all data, Please! \nQuantity >0" ("message") -> [w2109]
              tunnel: [TRUE ("Key Focus")] -> w2105
              tunnel: w2105 -> [w2111]
              tunnel: [w2111] -> w2104
              tunnel: w2104 -> [w2112]
              frame #0 {
                n261 = One Button Dialog(message=w2109) -> ()  [unwired: 1 in, 1 out]
              }
              frame #1 {
                n262 = Wait (ms)(milliseconds to wait=u32 10) -> ()  [unwired: 1 out]
              }
              frame #2 {
                n263 = property on="QR Code (F3)" class="Str"("Key Focus"=w2112) -> ()  [unwired: 2 in, 2 out]
              }
            }
          }
        }
        n264 = local write "BUTTON_INPUT"(w1406) -> ()
        n265 = case shown="False" w1408 {
          frame False {
            n266 = flat-sequence {
              tunnel: "" -> [w1433]
              tunnel: [w1433] -> w1430
              tunnel: w1430 -> [w1434]
              frame #0 {
                n267 = Wait (ms)(milliseconds to wait=u32 10) -> ()  [unwired: 1 out]
              }
              frame #1 {
                n268 = local write "Maker"(w1434) -> ()
                n269 = local write "Unit 2"(w1434) -> ()
                n270 = invoke on="Invoice Date" class="AbsTime (strict)" method="Reinit To Default"() -> ()  [unwired: 3 in, 3 out]
                n271 = local write "Quantity (F2)"(0.0 ("Quantity")) -> ()
                n272 = property on="QR Code (F3)" class="Str"("Key Focus"=TRUE) -> ()  [unwired: 2 in, 2 out]
                n273 = local write "QR Code (F3)"(w1434) -> ()
                n274 = local write "Invoice No."(w1434) -> ()
                n275 = local write "Product"(w1434) -> ()
                n276 = local write "Maker Code"(w1434) -> ()
                n277 = local write "Part Name"(w1434) -> ()
                n278 = local write "Lot Maker"(w1434) -> ()
                n279 = local write "Location"(w1434) -> ()
                n280 = local write "Item Code"(w1434) -> ()
                n281 = property on="Excle Path" class="Path"("Visible"=FALSE) -> ()  [unwired: 2 in, 2 out]
              }
            }
          }
          frame True {
          }
        }
      }
      event "Print Button": Value Change {
        n282 = event-data() -> ("OldVal"=w2113:bool)  [unwired: 1 in, 5 out]
        n283 = flat-sequence {
          tunnel: [w2139] -> w2114
          tunnel: w2113 -> [w2139]
          frame #0 {
            n284 = Wait (ms)(milliseconds to wait=u32 500) -> ()  [unwired: 1 out]
          }
        }
        n285 = local read "BALANCE_PRINT"() -> (w2115:bool)
        n286 = case shown="True" w2115 {
          tunnel: [w2140 w2141] -> w2117
          frame False {
            n287 = local read "Quantity (F2)"() -> (w2140:dbl)
          }
          frame True {
            n288 = property on="Table" class="Tbl (strict)"() -> ("Index Values"=w2146:T3)  [unwired: 2 in, 2 out]
            n289 = Unbundle By Name(w2146) -> ("Row"=w2144:u32)
            n290 = local read "Table"() -> (w2145:string[][])
            n291 = Index Array(array=w2145, index (row)=w2144, index (col)=9 ("disabled index (col)")) -> (element=w2142:string)
            n292 = Decimal String To Number(string=w2142) -> (number=w2141:i32)  [unwired: 2 in, 1 out]
          }
        }
        n293 = local write "Print Button"(w2114) -> ()
        n294 = local read "Invoice Date"() -> (w2127:timestamp)
        n295 = local read "Maker Code"() -> (w2116:string)
        n296 = local read "Invoice No."() -> (w2121:string)
        n297 = local read "Item Code"() -> (w2124:string)
        n298 = local read "Product"() -> (w2120:string)
        n299 = local read "ECODE"() -> (w2123:string)
        n300 = local read "Maker"() -> (w2118:string)
        n301 = local read "Unit 2"() -> (w2119:string)
        n302 = Less?(x=w2127, y=timestamp(3345170400 s since 1904-01-01)) -> (x < y?=w2133:bool)
        n303 = Empty String/Path?(string/path=w2124) -> (empty?=w2129:bool)
        n304 = Empty String/Path?(string/path=w2121) -> (empty?=w2131:bool)
        n305 = Empty String/Path?(string/path=w2123) -> (empty?=w2130:bool)
        n306 = Empty String/Path?(string/path=w2120) -> (empty?=w2132:bool)
        n307 = Empty String/Path?(string/path=w2118) -> (empty?=w2135:bool)
        n308 = Empty String/Path?(string/path=w2119) -> (empty?=w2134:bool)
        n309 = Empty String/Path?(string/path=w2116) -> (empty?=w2137:bool)
        n310 = Less Or Equal To 0?(x=w2117) -> (x <= 0?=w2136:bool)
        n311 = Compound Arithmetic op=OR(w2129, w2130, w2131, w2132, w2133, w2134, w2135, w2136, w2137) -> (w2125:bool)
        n312 = Format Date/Time String(time format string (%c)="%d/%m/%Y", seconds (now)=w2127) -> (date/time string=w2122:string)  [unwired: 1 in]
        n313 = case shown="False" w2125 {
          tunnel: ["" ""] -> _
          tunnel: w2124 -> [w2156 _]
          tunnel: w2123 -> [w2148 _]
          tunnel: w2122 -> [w2155 _]
          tunnel: w2121 -> [w2154 _]
          tunnel: w2120 -> [w2150 _]
          tunnel: w2119 -> [w2161 _]
          tunnel: w2118 -> [w2153 _]
          tunnel: w2117 -> [w2160 _]
          tunnel: w2116 -> [w2152 _]
          frame False {
            w2166 = "\\" ("string")
            n314 = local read "Lot Maker"() -> (w2159:string)
            n315 = Number To Decimal String(number=w2160) -> (decimal integer string=w2164:string)  [unwired: 1 in]
            n316 = call <vilib>:"Space Constant.vi"() -> ("String"=w2165:string)
            n317 = local read "Location"() -> (w2151:string)
            n318 = Concatenate Strings(w2156, w2166, w2155, w2166, w2154, w2166, w2164, w2166, w2159) -> (w2157:string)
            n319 = Concatenate Strings(w2164, w2165, w2161) -> (w2149:string)
            n320 = Bundle By Name(cluster=T8 {"QR_code Text"="", "Lot Maker"="", "Item Code (F3)"="", "date/time string"="", "Invoice No."="", "Maker"="", "Part No.(F2) "="", "Location"="", "Product"="", "Qty"="", "ECODE"=""} ("output cluster"), "QR_code Text"=w2157, "Lot Maker"=w2156, "Item Code (F3)"=w2156, "date/time string"=w2155, "Invoice No."=w2154, "Maker"=w2153, "Part No.(F2)"=w2152, "Location"=w2151, "Product"=w2150, "Qty"=w2149, "ECODE"=w2148) -> (w2147:T8)
            n321 = call "QR Code Generator Main.vi"("Print Button"=TRUE, "output cluster"=w2147) -> ()  [unwired: 10 in]
          }
          frame True {
            n322 = One Button Dialog(message="Full fill Data, Please") -> ()  [unwired: 1 in, 1 out]
          }
        }
      }
      event "BUTTON_EXIT": Value Change {
        n323 = event-data() -> ()  [unwired: 1 in, 6 out]
      }
    }
  }
